vi "Set Initialization Data - Oscilloscope.vi"(8 "error in":errorcluster, 11 "TopUI in":refnum<class "TopUI.lvclass">) -> (0 "error out":errorcluster, 3 "TopUI out":refnum<class "TopUI.lvclass">)   [LabVIEW 2018, in "TopUI.lvclass"]
doc: "In this VI you can set the initialization data of a statically-linked subWorker."
uses:
  TopUI.lvclass
  Oscilloscope/Response Cases.ctl
  Oscilloscope/Oscilloscope.lvclass
  Oscilloscope/Initialization Data.ctl
  <vilib>/addons/_Workers/Library/Case Label.ctl
  <vilib>/addons/_Workers/Library/Workers.lvlib
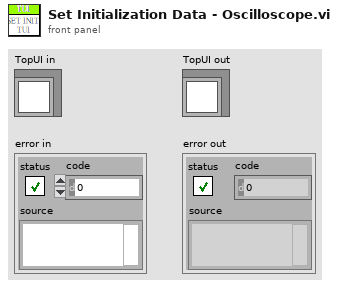
[diagram p1: front panel]
types:
  T1 = typedef "Oscilloscope.lvclass/Initialization Data.ctl" = cluster{"Response Cases":T2}
  T2 = typedef "Oscilloscope.lvclass/Response Cases.ctl" = cluster{"Placeholder - Can be deleted":string, "WaveformDataRuturn":T3}
  T3 = typedef "Workers.lvlib/Case Label.ctl" = string
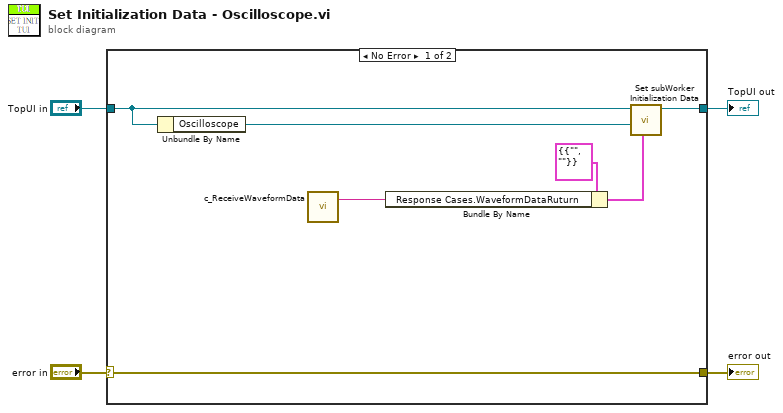
[diagram p0: block diagram]
diagram:
  n1 = case shown="No Error" "error in" {
    selector: "error in" -> [w11 w13]
    tunnel: [w11 w13] -> w3
    tunnel: [w9 w12] -> w2
    tunnel: "TopUI in" -> [w8 w12]
    frame No Error {
      n2 = Unbundle By Name(w8) -> ("Oscilloscope"=w10:refnum<class "Oscilloscope.lvclass">)
      n3 = call "c_ReceiveWaveformData.vi"() -> ("Case Label"=w5:T3)  [unwired: 1 in]
      n4 = Bundle By Name(cluster=T1 {"Response Cases"={"Placeholder - Can be deleted"="", "WaveformDataRuturn"=""}} ("Initialization Data"), "Response Cases.WaveformDataRuturn"=w5) -> (w6:T1)
      n5 = call-dynamic "Set subWorker Initialization Data.vi"("Initialization Data"=w6, "subWorker"=w10, "Worker"=w8) -> ("Worker out"=w9:refnum<class "TopUI.lvclass">)  [unwired: 8 in]
    }
    frame Error {
    }
  }
  "error out" <- w3
  "TopUI out" <- w2
